vi "WILT Initialize Agilent Channels Wilt.vi"(0 "Agilent Number":i32, 1 "VISA Resource Name":refnum<visa-resource-name>, 5 "Data Array":T1, 11 "error in (no error)":errorcluster) -> (4 "Number of Read Channels":i32, 15 "error out":errorcluster)   [LabVIEW 2016]
uses:
  Type Definitions/WILT Agilent Data Cluster.ctl
  Type Definitions/WILT Agilent Channel Definition.ctl
  Drivers/Agilent 34972/Agilent 34970.lvlib
panel:
  in  "Debug":bool
  in  "Debug":T1=[{"Channel"="(3_0_L1Current)101", "Station"="1", "Label"="L1 Current", "Agilent Station"="1", "Data"=0.0}, {"Channel"="(3_0_L2Current)102", "Station"="1", "Label"="L2 Current", "Agilent Station"="1", "Data"=0.0}, {"Channel"="(3_0_L1Current)103", "Station"="2", "Label"="L1 Current", "Agilent Station"="1", "Data"=0.0}, {"Channel"="(3_0_L2Current)104", "Station"="2", "Label"="L2 Current", "Agilent Station"="1", "Data"=0.0}, {"Channel"="(3_0_L1Current)105", "Station"="3", "Label"="L1 Current", "Agilent Station"="1", "Data"=0.0}, {"Channel"="(3_0_L2Current)106", "Station"="3", "Label"="L2 Current", "Agilent Station"="1", "Data"=0.0}, {"Channel"="(3_0_L1Current)107", "Station"="4", "Label"="L1 Current", "Agilent Station"="1", "Data"=0.0}, {"Channel"="(3_0_L2Current)108", "Station"="4", "Label"="L2 Current", "Agilent Station"="1", "Data"=0.0}, {"Channel"="(3_0_L1Current)109", "Station"="5", "Label"="L1 Current", "Agilent Station"="1", "Data"=0.0}, {"Channel"="(3_0_L2Current)110", "Station"="5", "Label"="L2 Current", "Agilent Station"="1", "Data"=0.0}, {"Channel"="(3_0_L1Current)111", "Station"="6", "Label"="L1 Current", "Agilent Station"="1", "Data"=0.0}, {"Channel"="(3_0_L2Current)112", "Station"="6", "Label"="L2 Current", "Agilent Station"="1", "Data"=0.0}, {"Channel"="(3_0_L1Current)113", "Station"="7", "Label"="L1 Current", "Agilent Station"="1", "Data"=0.0}, {"Channel"="(3_0_L2Current)114", "Station"="7", "Label"="L2 Current", "Agilent Station"="1", "Data"=0.0}, {"Channel"="(3_0_L1Current)115", "Station"="8", "Label"="L1 Current", "Agilent Station"="1", "Data"=0.0}, {"Channel"="(3_0_L2Current)116", "Station"="8", "Label"="L2 Current", "Agilent Station"="1", "Data"=0.0}, {"Channel"="(3_0_L1Current)201", "Station"="9", "Label"="L1 Current", "Agilent Station"="1", "Data"=0.0}, {"Channel"="(3_0_L2Current)202", "Station"="9", "Label"="L2 Current", "Agilent Station"="1", "Data"=0.0}, {"Channel"="(3_0_L1Current)203", "Station"="10", "Label"="L1 Current", "Agilent Station"="1", "Data"=0.0}, {"Channel"="(3_0_L2Current)204", "Station"="10", "Label"="L2 Current", "Agilent Station"="1", "Data"=0.0}, {"Channel"="(3_0_L1Current)205", "Station"="11", "Label"="L1 Current", "Agilent Station"="1", "Data"=0.0}, {"Channel"="(3_0_L2Current)206", "Station"="11", "Label"="L2 Current", "Agilent Station"="1", "Data"=0.0}, {"Channel"="(3_0_L1Current)207", "Station"="12", "Label"="L1 Current", "Agilent Station"="1", "Data"=0.0}, {"Channel"="(3_0_L2Current)208", "Station"="12", "Label"="L2 Current", "Agilent Station"="1", "Data"=0.0}, {"Channel"="(3_0_L1Current)209", "Station"="13", "Label"="L1 Current", "Agilent Station"="1", "Data"=0.0}, {"Channel"="(3_0_L2Current)210", "Station"="13", "Label"="L2 Current", "Agilent Station"="1", "Data"=0.0}, {"Channel"="(3_0_L1Current)211", "Station"="14", "Label"="L1 Current", "Agilent Station"="1", "Data"=0.0}, {"Channel"="(3_0_L2Current)212", "Station"="14", "Label"="L2 Current", "Agilent Station"="1", "Data"=0.0}, {"Channel"="(3_0_L1Current)213", "Station"="15", "Label"="L1 Current", "Agilent Station"="1", "Data"=0.0}, {"Channel"="(3_0_L2Current)214", "Station"="15", "Label"="L2 Current", "Agilent Station"="1", "Data"=0.0}, {"Channel"="(3_0_L1Current)215", "Station"="16", "Label"="L1 Current", "Agilent Station"="1", "Data"=0.0}, {"Channel"="(3_0_L2Current)216", "Station"="16", "Label"="L2 Current", "Agilent Station"="1", "Data"=0.0}, {"Channel"="(3_0_L1Current)301", "Station"="17", "Label"="L1 Current", "Agilent Station"="1", "Data"=0.0}, {"Channel"="(3_0_L2Current)302", "Station"="17", "Label"="L2 Current", "Agilent Station"="1", "Data"=0.0}, {"Channel"="(3_0_L1Current)303", "Station"="18", "Label"="L1 Current", "Agilent Station"="1", "Data"=0.0}, {"Channel"="(3_0_L2Current)304", "Station"="18", "Label"="L2 Current", "Agilent Station"="1", "Data"=0.0}, {"Channel"="(3_0_L1Current)305", "Station"="19", "Label"="L1 Current", "Agilent Station"="1", "Data"=0.0}, {"Channel"="(3_0_L2Current)306", "Station"="19", "Label"="L2 Current", "Agilent Station"="1", "Data"=0.0}, {"Channel"="(3_0_L1Current)307", "Station"="20", "Label"="L1 Current", "Agilent Station"="1", "Data"=0.0}, {"Channel"="(3_0_L2Current)308", "Station"="20", "Label"="L2 Current", "Agilent Station"="1", "Data"=0.0}, {"Channel"="(3_0_L1Current)309", "Station"="21", "Label"="L1 Current", "Agilent Station"="1", "Data"=0.0}, {"Channel"="(3_0_L2Current)310", "Station"="21", "Label"="L2 Current", "Agilent Station"="1", "Data"=0.0}, {"Channel"="(3_0_L1Current)311", "Station"="22", "Label"="L1 Current", "Agilent Station"="1", "Data"=0.0}, {"Channel"="(3_0_L2Current)312", "Station"="22", "Label"="L2 Current", "Agilent Station"="1", "Data"=0.0}, {"Channel"="(3_0_L1Current)313", "Station"="23", "Label"="L1 Current", "Agilent Station"="1", "Data"=0.0}, {"Channel"="(3_0_L2Current)314", "Station"="23", "Label"="L2 Current", "Agilent Station"="1", "Data"=0.0}, {"Channel"="(3_0_L1Current)315", "Station"="24", "Label"="L1 Current", "Agilent Station"="1", "Data"=0.0}, {"Channel"="(3_0_L2Current)316", "Station"="24", "Label"="L2 Current", "Agilent Station"="1", "Data"=0.0}, {"Channel"="(3_0_L1Current)101", "Station"="25", "Label"="L1 Current", "Agilent Station"="2", "Data"=0.0}, {"Channel"="(3_0_L2Current)102", "Station"="25", "Label"="L2 Current", "Agilent Station"="2", "Data"=0.0}, {"Channel"="(3_0_L1Current)103", "Station"="26", "Label"="L1 Current", "Agilent Station"="2", "Data"=0.0}, {"Channel"="(3_0_L2Current)104", "Station"="26", "Label"="L2 Current", "Agilent Station"="2", "Data"=0.0}, {"Channel"="(3_0_L1Current)105", "Station"="27", "Label"="L1 Current", "Agilent Station"="2", "Data"=0.0}, {"Channel"="(3_0_L2Current)106", "Station"="27", "Label"="L2 Current", "Agilent Station"="2", "Data"=0.0}, {"Channel"="(3_0_L1Current)107", "Station"="28", "Label"="L1 Current", "Agilent Station"="2", "Data"=0.0}, {"Channel"="(3_0_L2Current)108", "Station"="28", "Label"="L2 Current", "Agilent Station"="2", "Data"=0.0}, {"Channel"="(3_0_L1Current)109", "Station"="29", "Label"="L1 Current", "Agilent Station"="2", "Data"=0.0}, {"Channel"="(3_0_L2Current)110", "Station"="29", "Label"="L2 Current", "Agilent Station"="2", "Data"=0.0}, {"Channel"="(3_0_L1Current)111", "Station"="30", "Label"="L1 Current", "Agilent Station"="2", "Data"=0.0}, {"Channel"="(3_0_L2Current)112", "Station"="30", "Label"="L2 Current", "Agilent Station"="2", "Data"=0.0}, {"Channel"="(3_0_L1Current)113", "Station"="31", "Label"="L1 Current", "Agilent Station"="2", "Data"=0.0}, {"Channel"="(3_0_L2Current)114", "Station"="31", "Label"="L2 Current", "Agilent Station"="2", "Data"=0.0}, {"Channel"="(3_0_L1Current)115", "Station"="32", "Label"="L1 Current", "Agilent Station"="2", "Data"=0.0}, {"Channel"="(3_0_L2Current)116", "Station"="32", "Label"="L2 Current", "Agilent Station"="2", "Data"=0.0}, {"Channel"="(30_0_Volts)201", "Station"="5", "Label"="Volts", "Agilent Station"="2", "Data"=0.0}, {"Channel"="(30_0_Volts)202", "Station"="6", "Label"="Volts", "Agilent Station"="2", "Data"=0.0}, {"Channel"="(30_0_Volts)203", "Station"="7", "Label"="Volts", "Agilent Station"="2", "Data"=0.0}, {"Channel"="(30_0_Volts)204", "Station"="8", "Label"="Volts", "Agilent Station"="2", "Data"=0.0}, {"Channel"="(30_0_Volts)205", "Station"="9", "Label"="Volts", "Agilent Station"="2", "Data"=0.0}, {"Channel"="(30_0_Volts)206", "Station"="10", "Label"="Volts", "Agilent Station"="2", "Data"=0.0}, {"Channel"="(30_0_Volts)207", "Station"="11", "Label"="Volts", "Agilent Station"="2", "Data"=0.0}, {"Channel"="(30_0_Volts)208", "Station"="12", "Label"="Volts", "Agilent Station"="2", "Data"=0.0}, {"Channel"="(30_0_Volts)209", "Station"="13", "Label"="Volts", "Agilent Station"="2", "Data"=0.0}, {"Channel"="(30_0_Volts)210", "Station"="14", "Label"="Volts", "Agilent Station"="2", "Data"=0.0}, {"Channel"="(30_0_Volts)211", "Station"="21", "Label"="Volts", "Agilent Station"="2", "Data"=0.0}, {"Channel"="(30_0_Volts)211", "Station"="22", "Label"="Volts", "Agilent Station"="2", "Data"=0.0}, {"Channel"="(30_0_Volts)211", "Station"="23", "Label"="Volts", "Agilent Station"="2", "Data"=0.0}, {"Channel"="(30_0_Volts)212", "Station"="24", "Label"="Volts", "Agilent Station"="2", "Data"=0.0}, {"Channel"="(30_0_Volts)212", "Station"="25", "Label"="Volts", "Agilent Station"="2", "Data"=0.0}, {"Channel"="(30_0_Volts)212", "Station"="26", "Label"="Volts", "Agilent Station"="2", "Data"=0.0}, {"Channel"="(30_0_Volts)213", "Station"="27", "Label"="Volts", "Agilent Station"="2", "Data"=0.0}, {"Channel"="(30_0_Volts)213", "Station"="28", "Label"="Volts", "Agilent Station"="2", "Data"=0.0}, {"Channel"="(30_0_Volts)213", "Station"="29", "Label"="Volts", "Agilent Station"="2", "Data"=0.0}, {"Channel"="(30_0_Volts)214", "Station"="30", "Label"="Volts", "Agilent Station"="2", "Data"=0.0}, {"Channel"="(30_0_Volts)214", "Station"="31", "Label"="Volts", "Agilent Station"="2", "Data"=0.0}, {"Channel"="(30_0_Volts)214", "Station"="32", "Label"="Volts", "Agilent Station"="2", "Data"=0.0}, {"Channel"="(30_0_Volts)215", "Station"="15", "Label"="Volts", "Agilent Station"="2", "Data"=0.0}, {"Channel"="(30_0_Volts)216", "Station"="16", "Label"="Volts", "Agilent Station"="2", "Data"=0.0}, {"Channel"="201", "Station"="1", "Label"="Temperature", "Agilent Station"="3", "Data"=0.0}, {"Channel"="202", "Station"="2", "Label"="Temperature", "Agilent Station"="3", "Data"=0.0}, {"Channel"="203", "Station"="3", "Label"="Temperature", "Agilent Station"="3", "Data"=0.0}, {"Channel"="204", "Station"="4", "Label"="Temperature", "Agilent Station"="3", "Data"=0.0}, {"Channel"="205", "Station"="5", "Label"="Temperature", "Agilent Station"="3", "Data"=0.0}, {"Channel"="206", "Station"="6", "Label"="Temperature", "Agilent Station"="3", "Data"=0.0}, {"Channel"="207", "Station"="7", "Label"="Temperature", "Agilent Station"="3", "Data"=0.0}, {"Channel"="208", "Station"="8", "Label"="Temperature", "Agilent Station"="3", "Data"=0.0}, {"Channel"="209", "Station"="9", "Label"="Temperature", "Agilent Station"="3", "Data"=0.0}, {"Channel"="210", "Station"="10", "Label"="Temperature", "Agilent Station"="3", "Data"=0.0}, {"Channel"="211", "Station"="11", "Label"="Temperature", "Agilent Station"="3", "Data"=0.0}, {"Channel"="212", "Station"="12", "Label"="Temperature", "Agilent Station"="3", "Data"=0.0}, {"Channel"="213", "Station"="13", "Label"="Temperature", "Agilent Station"="3", "Data"=0.0}, {"Channel"="214", "Station"="14", "Label"="Temperature", "Agilent Station"="3", "Data"=0.0}, {"Channel"="215", "Station"="15", "Label"="Temperature", "Agilent Station"="3", "Data"=0.0}, {"Channel"="216", "Station"="16", "Label"="Temperature", "Agilent Station"="3", "Data"=0.0}, {"Channel"="217", "Station"="17", "Label"="Temperature", "Agilent Station"="3", "Data"=0.0}, {"Channel"="218", "Station"="18", "Label"="Temperature", "Agilent Station"="3", "Data"=0.0}, {"Channel"="219", "Station"="19", "Label"="Temperature", "Agilent Station"="3", "Data"=0.0}, {"Channel"="220", "Station"="20", "Label"="Temperature", "Agilent Station"="3", "Data"=0.0}, {"Channel"="301", "Station"="21", "Label"="Temperature", "Agilent Station"="3", "Data"=0.0}, {"Channel"="302", "Station"="22", "Label"="Temperature", "Agilent Station"="3", "Data"=0.0}, {"Channel"="303", "Station"="23", "Label"="Temperature", "Agilent Station"="3", "Data"=0.0}, {"Channel"="304", "Station"="24", "Label"="Temperature", "Agilent Station"="3", "Data"=0.0}, {"Channel"="305", "Station"="25", "Label"="Temperature", "Agilent Station"="3", "Data"=0.0}, {"Channel"="306", "Station"="26", "Label"="Temperature", "Agilent Station"="3", "Data"=0.0}, {"Channel"="307", "Station"="27", "Label"="Temperature", "Agilent Station"="3", "Data"=0.0}, {"Channel"="308", "Station"="28", "Label"="Temperature", "Agilent Station"="3", "Data"=0.0}, {"Channel"="309", "Station"="29", "Label"="Temperature", "Agilent Station"="3", "Data"=0.0}, {"Channel"="310", "Station"="30", "Label"="Temperature", "Agilent Station"="3", "Data"=0.0}, {"Channel"="311", "Station"="31", "Label"="Temperature", "Agilent Station"="3", "Data"=0.0}, {"Channel"="312", "Station"="32", "Label"="Temperature", "Agilent Station"="3", "Data"=0.0}, {"Channel"="(30_0_Volts)313", "Station"="1", "Label"="Volts", "Agilent Station"="3", "Data"=0.0}, {"Channel"="(30_0_Volts)314", "Station"="2", "Label"="Volts", "Agilent Station"="3", "Data"=0.0}, {"Channel"="(30_0_Volts)315", "Station"="3", "Label"="Volts", "Agilent Station"="3", "Data"=0.0}, {"Channel"="(30_0_Volts)316", "Station"="4", "Label"="Volts", "Agilent Station"="3", "Data"=0.0}, {"Channel"="(3_0_L1Current)101", "Station"="33", "Label"="L1 Current", "Agilent Station"="4", "Data"=0.0}, {"Channel"="(3_0_L2Current)102", "Station"="33", "Label"="L2 Current", "Agilent Station"="4", "Data"=0.0}, {"Channel"="(3_0_L1Current)103", "Station"="34", "Label"="L1 Current", "Agilent Station"="4", "Data"=0.0}, {"Channel"="(3_0_L2Current)104", "Station"="34", "Label"="L2 Current", "Agilent Station"="4", "Data"=0.0}, {"Channel"="(3_0_L1Current)105", "Station"="35", "Label"="L1 Current", "Agilent Station"="4", "Data"=0.0}, {"Channel"="(3_0_L2Current)106", "Station"="35", "Label"="L2 Current", "Agilent Station"="4", "Data"=0.0}, {"Channel"="(3_0_L1Current)107", "Station"="36", "Label"="L1 Current", "Agilent Station"="4", "Data"=0.0}, {"Channel"="(3_0_L2Current)108", "Station"="36", "Label"="L2 Current", "Agilent Station"="4", "Data"=0.0}, {"Channel"="(3_0_L1Current)109", "Station"="37", "Label"="L1 Current", "Agilent Station"="4", "Data"=0.0}, {"Channel"="(3_0_L2Current)110", "Station"="37", "Label"="L2 Current", "Agilent Station"="4", "Data"=0.0}, {"Channel"="(3_0_L1Current)111", "Station"="38", "Label"="L1 Current", "Agilent Station"="4", "Data"=0.0}, {"Channel"="(3_0_L2Current)112", "Station"="38", "Label"="L2 Current", "Agilent Station"="4", "Data"=0.0}, {"Channel"="(3_0_L1Current)113", "Station"="39", "Label"="L1 Current", "Agilent Station"="4", "Data"=0.0}, {"Channel"="(3_0_L2Current)114", "Station"="39", "Label"="L2 Current", "Agilent Station"="4", "Data"=0.0}, {"Channel"="(3_0_L1Current)115", "Station"="40", "Label"="L1 Current", "Agilent Station"="4", "Data"=0.0}, {"Channel"="(3_0_L2Current)116", "Station"="40", "Label"="L2 Current", "Agilent Station"="4", "Data"=0.0}, {"Channel"="(3_0_L1Current)201", "Station"="41", "Label"="L1 Current", "Agilent Station"="4", "Data"=0.0}, {"Channel"="(3_0_L2Current)202", "Station"="41", "Label"="L2 Current", "Agilent Station"="4", "Data"=0.0}, {"Channel"="(3_0_L1Current)203", "Station"="42", "Label"="L1 Current", "Agilent Station"="4", "Data"=0.0}, {"Channel"="(3_0_L2Current)204", "Station"="42", "Label"="L2 Current", "Agilent Station"="4", "Data"=0.0}, {"Channel"="(3_0_L1Current)205", "Station"="43", "Label"="L1 Current", "Agilent Station"="4", "Data"=0.0}, {"Channel"="(3_0_L2Current)206", "Station"="43", "Label"="L2 Current", "Agilent Station"="4", "Data"=0.0}, {"Channel"="(3_0_L1Current)207", "Station"="44", "Label"="L1 Current", "Agilent Station"="4", "Data"=0.0}, {"Channel"="(3_0_L2Current)208", "Station"="44", "Label"="L2 Current", "Agilent Station"="4", "Data"=0.0}, {"Channel"="(3_0_L1Current)209", "Station"="45", "Label"="L1 Current", "Agilent Station"="4", "Data"=0.0}, {"Channel"="(3_0_L2Current)210", "Station"="45", "Label"="L2 Current", "Agilent Station"="4", "Data"=0.0}, {"Channel"="(3_0_L1Current)211", "Station"="46", "Label"="L1 Current", "Agilent Station"="4", "Data"=0.0}, {"Channel"="(3_0_L2Current)212", "Station"="46", "Label"="L2 Current", "Agilent Station"="4", "Data"=0.0}, {"Channel"="(3_0_L1Current)213", "Station"="47", "Label"="L1 Current", "Agilent Station"="4", "Data"=0.0}, {"Channel"="(3_0_L2Current)214", "Station"="47", "Label"="L2 Current", "Agilent Station"="4", "Data"=0.0}, {"Channel"="(3_0_L1Current)215", "Station"="48", "Label"="L1 Current", "Agilent Station"="4", "Data"=0.0}, {"Channel"="(3_0_L2Current)216", "Station"="48", "Label"="L2 Current", "Agilent Station"="4", "Data"=0.0}, {"Channel"="(3_0_L1Current)301", "Station"="49", "Label"="L1 Current", "Agilent Station"="4", "Data"=0.0}, {"Channel"="(3_0_L2Current)302", "Station"="49", "Label"="L2 Current", "Agilent Station"="4", "Data"=0.0}, {"Channel"="(3_0_L1Current)303", "Station"="50", "Label"="L1 Current", "Agilent Station"="4", "Data"=0.0}, {"Channel"="(3_0_L2Current)304", "Station"="50", "Label"="L2 Current", "Agilent Station"="4", "Data"=0.0}, {"Channel"="(3_0_L1Current)305", "Station"="51", "Label"="L1 Current", "Agilent Station"="4", "Data"=0.0}, {"Channel"="(3_0_L2Current)306", "Station"="51", "Label"="L2 Current", "Agilent Station"="4", "Data"=0.0}, {"Channel"="(3_0_L1Current)307", "Station"="52", "Label"="L1 Current", "Agilent Station"="4", "Data"=0.0}, {"Channel"="(3_0_L2Current)308", "Station"="52", "Label"="L2 Current", "Agilent Station"="4", "Data"=0.0}, {"Channel"="(3_0_L1Current)309", "Station"="53", "Label"="L1 Current", "Agilent Station"="4", "Data"=0.0}, {"Channel"="(3_0_L2Current)310", "Station"="53", "Label"="L2 Current", "Agilent Station"="4", "Data"=0.0}, {"Channel"="(3_0_L1Current)311", "Station"="54", "Label"="L1 Current", "Agilent Station"="4", "Data"=0.0}, {"Channel"="(3_0_L2Current)312", "Station"="54", "Label"="L2 Current", "Agilent Station"="4", "Data"=0.0}, {"Channel"="(3_0_L1Current)313", "Station"="55", "Label"="L1 Current", "Agilent Station"="4", "Data"=0.0}, {"Channel"="(3_0_L2Current)314", "Station"="55", "Label"="L2 Current", "Agilent Station"="4", "Data"=0.0}, {"Channel"="(3_0_L1Current)315", "Station"="56", "Label"="L1 Current", "Agilent Station"="4", "Data"=0.0}, {"Channel"="(3_0_L2Current)316", "Station"="56", "Label"="L2 Current", "Agilent Station"="4", "Data"=0.0}, {"Channel"="101", "Station"="33", "Label"="Temperature", "Agilent Station"="6", "Data"=0.0}, {"Channel"="102", "Station"="34", "Label"="Temperature", "Agilent Station"="6", "Data"=0.0}, {"Channel"="103", "Station"="35", "Label"="Temperature", "Agilent Station"="6", "Data"=0.0}, {"Channel"="104", "Station"="36", "Label"="Temperature", "Agilent Station"="6", "Data"=0.0}, {"Channel"="105", "Station"="37", "Label"="Temperature", "Agilent Station"="6", "Data"=0.0}, {"Channel"="106", "Station"="38", "Label"="Temperature", "Agilent Station"="6", "Data"=0.0}, {"Channel"="107", "Station"="39", "Label"="Temperature", "Agilent Station"="6", "Data"=0.0}, {"Channel"="108", "Station"="40", "Label"="Temperature", "Agilent Station"="6", "Data"=0.0}, {"Channel"="109", "Station"="41", "Label"="Temperature", "Agilent Station"="6", "Data"=0.0}, {"Channel"="110", "Station"="42", "Label"="Temperature", "Agilent Station"="6", "Data"=0.0}, {"Channel"="111", "Station"="43", "Label"="Temperature", "Agilent Station"="6", "Data"=0.0}, {"Channel"="112", "Station"="44", "Label"="Temperature", "Agilent Station"="6", "Data"=0.0}, {"Channel"="113", "Station"="45", "Label"="Temperature", "Agilent Station"="6", "Data"=0.0}, {"Channel"="114", "Station"="46", "Label"="Temperature", "Agilent Station"="6", "Data"=0.0}, {"Channel"="115", "Station"="47", "Label"="Temperature", "Agilent Station"="6", "Data"=0.0}, {"Channel"="116", "Station"="48", "Label"="Temperature", "Agilent Station"="6", "Data"=0.0}, {"Channel"="117", "Station"="49", "Label"="Temperature", "Agilent Station"="6", "Data"=0.0}, {"Channel"="118", "Station"="50", "Label"="Temperature", "Agilent Station"="6", "Data"=0.0}, {"Channel"="119", "Station"="51", "Label"="Temperature", "Agilent Station"="6", "Data"=0.0}, {"Channel"="120", "Station"="52", "Label"="Temperature", "Agilent Station"="6", "Data"=0.0}, {"Channel"="201", "Station"="53", "Label"="Temperature", "Agilent Station"="6", "Data"=0.0}, {"Channel"="202", "Station"="54", "Label"="Temperature", "Agilent Station"="6", "Data"=0.0}, {"Channel"="203", "Station"="55", "Label"="Temperature", "Agilent Station"="6", "Data"=0.0}, {"Channel"="204", "Station"="56", "Label"="Temperature", "Agilent Station"="6", "Data"=0.0}, {"Channel"="(30_0_Volts)205", "Station"="33", "Label"="Volts", "Agilent Station"="6", "Data"=0.0}, {"Channel"="(30_0_Volts)205", "Station"="34", "Label"="Volts", "Agilent Station"="6", "Data"=0.0}, {"Channel"="(30_0_Volts)205", "Station"="35", "Label"="Volts", "Agilent Station"="6", "Data"=0.0}, {"Channel"="(30_0_Volts)206", "Station"="36", "Label"="Volts", "Agilent Station"="6", "Data"=0.0}, {"Channel"="(30_0_Volts)206", "Station"="37", "Label"="Volts", "Agilent Station"="6", "Data"=0.0}, {"Channel"="(30_0_Volts)206", "Station"="38", "Label"="Volts", "Agilent Station"="6", "Data"=0.0}, {"Channel"="(30_0_Volts)207", "Station"="39", "Label"="Volts", "Agilent Station"="6", "Data"=0.0}, {"Channel"="(30_0_Volts)207", "Station"="40", "Label"="Volts", "Agilent Station"="6", "Data"=0.0}, {"Channel"="(30_0_Volts)208", "Station"="42", "Label"="Volts", "Agilent Station"="6", "Data"=0.0}, {"Channel"="(30_0_Volts)208", "Station"="43", "Label"="Volts", "Agilent Station"="6", "Data"=0.0}, {"Channel"="(30_0_Volts)208", "Station"="44", "Label"="Volts", "Agilent Station"="6", "Data"=0.0}, {"Channel"="(30_0_Volts)209", "Station"="45", "Label"="Volts", "Agilent Station"="6", "Data"=0.0}, {"Channel"="(30_0_Volts)209", "Station"="46", "Label"="Volts", "Agilent Station"="6", "Data"=0.0}, {"Channel"="(30_0_Volts)209", "Station"="47", "Label"="Volts", "Agilent Station"="6", "Data"=0.0}, {"Channel"="(30_0_Volts)210", "Station"="45", "Label"="Volts (208)", "Agilent Station"="6", "Data"=0.0}, {"Channel"="211", "Station"="45", "Label"="SW (208)", "Agilent Station"="6", "Data"=0.0}, {"Channel"="(30_0_Volts)212", "Station"="48", "Label"="Volts", "Agilent Station"="6", "Data"=0.0}, {"Channel"="(30_0_Volts)212", "Station"="49", "Label"="Volts", "Agilent Station"="6", "Data"=0.0}, {"Channel"="(30_0_Volts)212", "Station"="50", "Label"="Volts", "Agilent Station"="6", "Data"=0.0}, {"Channel"="213", "Station"="48", "Label"="SW (208)", "Agilent Station"="6", "Data"=0.0}, {"Channel"="(30_0_Volts)214", "Station"="51", "Label"="Volts (208)", "Agilent Station"="6", "Data"=0.0}, {"Channel"="215", "Station"="51", "Label"="SW (208)", "Agilent Station"="6", "Data"=0.0}, {"Channel"="(30_0_Volts)216", "Station"="54", "Label"="Volts", "Agilent Station"="6", "Data"=0.0}, {"Channel"="(30_0_Volts)216", "Station"="55", "Label"="Volts", "Agilent Station"="6", "Data"=0.0}, {"Channel"="(30_0_Volts)216", "Station"="56", "Label"="Volts", "Agilent Station"="6", "Data"=0.0}, {"Channel"="(30_0_Volts)301", "Station"="17", "Label"="Volts", "Agilent Station"="6", "Data"=0.0}, {"Channel"="(30_0_Volts)302", "Station"="18", "Label"="Volts", "Agilent Station"="6", "Data"=0.0}, {"Channel"="(30_0_Volts)303", "Station"="19", "Label"="Volts", "Agilent Station"="6", "Data"=0.0}, {"Channel"="(30_0_Volts)304", "Station"="20", "Label"="Volts", "Agilent Station"="6", "Data"=0.0}, {"Channel"="(30_0_Volts)305", "Station"="51", "Label"="Volts", "Agilent Station"="6", "Data"=0.0}, {"Channel"="(30_0_Volts)305", "Station"="52", "Label"="Volts", "Agilent Station"="6", "Data"=0.0}, {"Channel"="(30_0_Volts)305", "Station"="53", "Label"="Volts", "Agilent Station"="6", "Data"=0.0}, {"Channel"="(30_0_Volts)306", "Station"="48", "Label"="Volts (208)", "Agilent Station"="6", "Data"=0.0}]
  out "Channel List":string
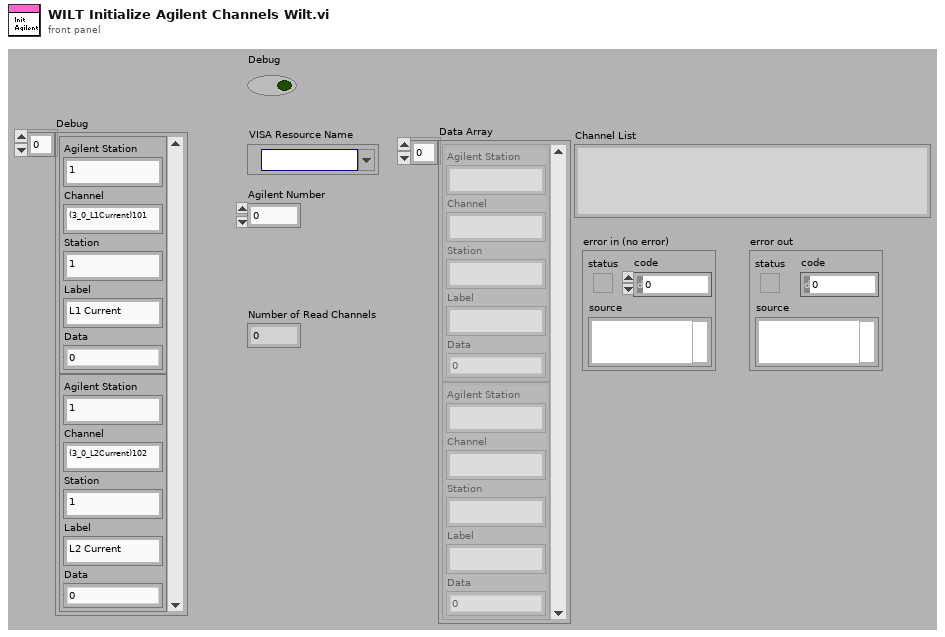
[diagram p1: front panel]
types:
  T1 = typedef "WILT Agilent Data Cluster.ctl" = T2[]
  T2 = typedef "WILT Agilent Channel Definition.ctl" = cluster{"Channel":string, "Station":string, "Label":string, "Agilent Station":string, "Data":dbl}
  T3 = enum16{"100 Ohm", "1 kOhm", "10 kOhm", "100 kOhm", "1 MOhm", "10 MOhm", "100 MOhm", "Minimum", "Maximum"}
  T4 = cluster{"Thermocouple Type (Last)":enum16{"B", "E", "J", "K", "N", "R", "S", "T", "Default (Last)"}, "TC Rjunction (2:Int)":enum16{"Fixed", "External", "Internal"}, "Fixed Rjunction Temp (0:Manual)":enum16{"Manual", "Minimum", "Maximum"}, "TC Auto Check? (F:Don't Check)":bool, "Rjunct Temp Value (0)":dbl}
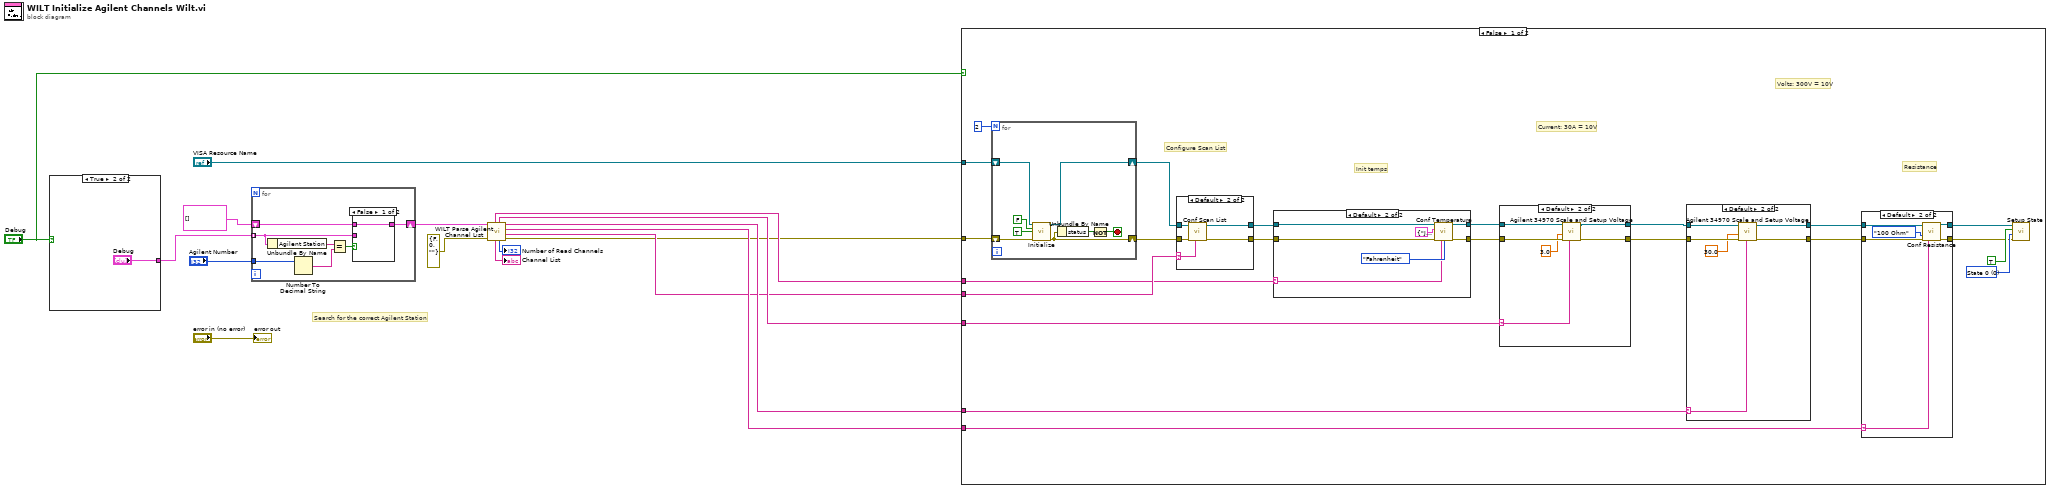
[diagram p0: block diagram]
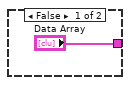
[diagram p2: hidden frame]
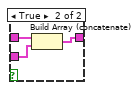
[diagram p9: hidden frame]
diagram:
  # "Search for the correct Agilent Station"
  n1 = case shown="True" "Debug" {
    tunnel: ["Data Array" "Debug"] -> w1
    frame False {
    }
    frame True {
    }
  }
  n2 = for {
    tunnel: w1 -> [w23] mode=indexing
    tunnel: "Agilent Number" -> [w19]
    shift-right: [w22] -> w15
    shift-left: T2[] [] -> [w21]
    n3 = Unbundle By Name(w23) -> ("Agilent Station"=w24:string)
    n4 = Number To Decimal String(number=w19) -> (decimal integer string=w25:string)  [unwired: 1 in]
    n5 = Equal?(x=w24, y=w25) -> (x = y?=w20:bool)
    n6 = case shown="False" w20 {
      tunnel: w23 -> [_ w29]
      tunnel: [w26 w28] -> w22
      tunnel: w21 -> [w26 w27]
      frame False {
      }
      frame True {
        n7 = Build Array (concatenate)(w27, w29) -> (w28:T2[])
      }
    }
  }
  n8 = call "WILT Parse Agilent Channel List.vi"("Error In"=errorcluster {"status"=FALSE, "code"=0, "source"=""} ("error out"), "Array"=w15) -> ("Error Out"=w4:errorcluster, "Configure Scan List"=w7:string, "Resistance"=w8:string, "Voltage"=w9:string, "Number of Read Channels"=→"Number of Read Channels":i32, "Current"=w10:string, "Channel List"=→"Channel List":string, "Temperature"=w5:string)  [unwired: 2 in]
  n9 = case shown="False" "Debug" {
    tunnel: w10 -> [w42 _]
    tunnel: w9 -> [w41 _]
    tunnel: w8 -> [w40 _]
    tunnel: w7 -> [w39 _]
    tunnel: w5 -> [w38 _]
    tunnel: w4 -> [w33 _]
    tunnel: "VISA Resource Name" -> [w32 _]
    frame False {
      w43 = u16 0 items=["State 0", "State 1", "State 2", "State 3", "State 4", "State 5", "Preset State"] ("Setup State (6:Preset)")
      # "Configure Scan List"
      # "Resistance"
      # "Volts: 300V = 10V"
      # "Current: 30A = 10V"
      # "Init temps"
      n10 = for {
        N: 2 -> [_]
        shift-right: [w58] -> w35
        shift-left: w32 -> [w59]
        shift-right: [w54] -> w34
        shift-left: w33 -> [w57]
        stop <- w53 stop-if-true
        n11 = call "Initialize.vi"("VISA Resource Name"=w59, "ID Query (T: Check)"=FALSE, "Reset (T: Reset)"=TRUE, "error in (no error)"=w57) -> ("VISA Resource Name Out"=w58:refnum<visa-resource-name>, "error out"=w54:errorcluster)  [unwired: 10 in]
        n12 = Unbundle By Name(w54) -> ("status"=w52:bool)
        n13 = Not(x=w52) -> (.not. x?=w53:bool)
      }
      n14 = case shown="Default" w39 {
        selector: w39 -> [_ w62]
        tunnel: w35 -> [w60 w66]
        tunnel: [w61 w65] -> w30
        tunnel: w34 -> [w61 w64]
        tunnel: [w60 w63] -> w31
        frame "" {
        }
        frame Default {
          n15 = call "Conf Scan List.vi"("Scan List (empty)"=w62, "error in (no error)"=w64, "VISA Resource Name"=w66) -> ("error out"=w65:errorcluster, "VISA Resource Name Out"=w63:refnum<visa-resource-name>)  [unwired: 6 in, 1 out]
        }
      }
      n16 = case shown="Default" w38 {
        selector: w38 -> [_ w94]
        tunnel: w31 -> [w91 w97]
        tunnel: [w92 w96] -> w51
        tunnel: w30 -> [w92 w95]
        tunnel: [w91 w93] -> w50
        frame "" {
        }
        frame Default {
          n17 = call "Conf Temperature.vi"("VISA Resource Name"=w97, "Thermocouple Configuration"=T4 {"Thermocouple Type (Last)"=enum."J", "TC Rjunction (2:Int)"=enum."Internal", "Fixed Rjunction Temp (0:Manual)"=enum."Manual", "TC Auto Check? (F:Don't Check)"=FALSE, "Rjunct Temp Value (0)"=0.0}, "error in (no error)"=w95, "Channel List(empty)"=w94, "Units (0:Celsius)"=enum16{"Celsius", "Fahrenheit", "Kelvin"}."Fahrenheit") -> ("VISA Resource Name Out"=w93:refnum<visa-resource-name>, "error out"=w96:errorcluster)  [unwired: 8 in, 1 out]
        }
      }
      n18 = case shown="Default" w42 {
        selector: w42 -> [_ w85]
        tunnel: w50 -> [w83 w88]
        tunnel: w51 -> [w84 w87]
        tunnel: [w84 w89] -> w48
        tunnel: [w83 w90] -> w49
        frame "" {
        }
        frame Default {
          n19 = call "Agilent 34970 Scale and Setup Voltage.vi"("Channel List"=w85, "error in (no error)"=w87, "Gain (1)"=3.0, "VISA Refnum in"=w88) -> ("error out"=w89:errorcluster, "VISA Refnum out"=w90:refnum<visa-resource-name>)  [unwired: 6 in]
        }
      }
      n20 = case shown="Default" w41 {
        selector: w41 -> [_ w77]
        tunnel: w49 -> [w75 w82]
        tunnel: w48 -> [w76 w81]
        tunnel: [w76 w80] -> w46
        tunnel: [w75 w79] -> w47
        frame "" {
        }
        frame Default {
          n21 = call "Agilent 34970 Scale and Setup Voltage.vi"("Channel List"=w77, "error in (no error)"=w81, "Gain (1)"=30.0, "VISA Refnum in"=w82) -> ("error out"=w80:errorcluster, "VISA Refnum out"=w79:refnum<visa-resource-name>)  [unwired: 6 in]
        }
      }
      n22 = case shown="Default" w40 {
        selector: w40 -> [_ w69]
        tunnel: w46 -> [w68 w74]
        tunnel: w47 -> [w67 w73]
        tunnel: [w68 w72] -> w37
        tunnel: [w67 w70] -> w36
        frame "" {
        }
        frame Default {
          n23 = call "Conf Resistance.vi"("VISA Resource Name"=w73, "Range (8:Maximum)"=T3."100 Ohm", "error in (no error)"=w74, "Channel List (empty)"=w69) -> ("VISA Resource Name Out"=w70:refnum<visa-resource-name>, "error out"=w72:errorcluster)  [unwired: 9 in, 1 out]
        }
      }
      n24 = call "Setup State.vi"("error in (no error)"=w37, "Setup State (6:Preset)"=w43, "Recall/Save (F=Recall)"=TRUE, "VISA Resource Name"=w36) -> ()  [unwired: 6 in, 2 out]
    }
    frame True {
    }
  }
  "error out" <- "error in (no error)"
